vi "Convert LIN frames to Trace log.vi"(11 "lin frames in":T1[](array[typedef]) {"event ID" format="%x"; "payload" format="%x"; "timestamp" format="%<%.7X\n%x>T"; "type" items=["LIN Data"=64, "LIN Bus Error"=65, "LIN No Response"=66, "Delay"=224, "Log Trigger"=225, "Start Trigger"=226]; "identifier" format="%x"}) -> (3 "trace out":string[][](array[string]))   [LabVIEW 2025, in "CAN-LIN Raw Bus Capture.lvclass"]
uses:
  CAN-LIN Raw Bus Capture.lvclass
  <vilib>/xnet/xnet.llb/XNET Frame LIN.ctl
  <vilib>/xnet/xnet.llb/XNET Frame Type LIN.ctl
  CAN-LIN Raw Bus Capture.lvclass/CAN-LIN Raw Bus Capture.ctl
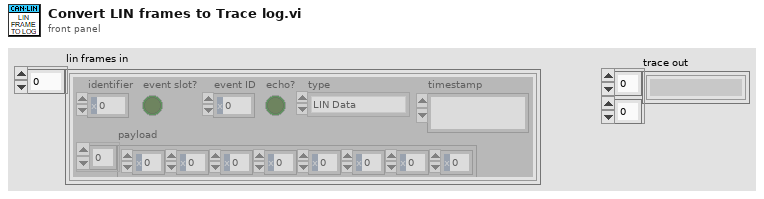
[diagram p1: front panel]
types:
  T1 = typedef "XNET Frame LIN.ctl" = cluster{"timestamp":timestamp, "payload":u8[], "identifier":u32, "type":T2, "event ID":u8, "event slot?":bool, "echo?":bool}
  T2 = typedef "XNET Frame Type LIN.ctl" = u8
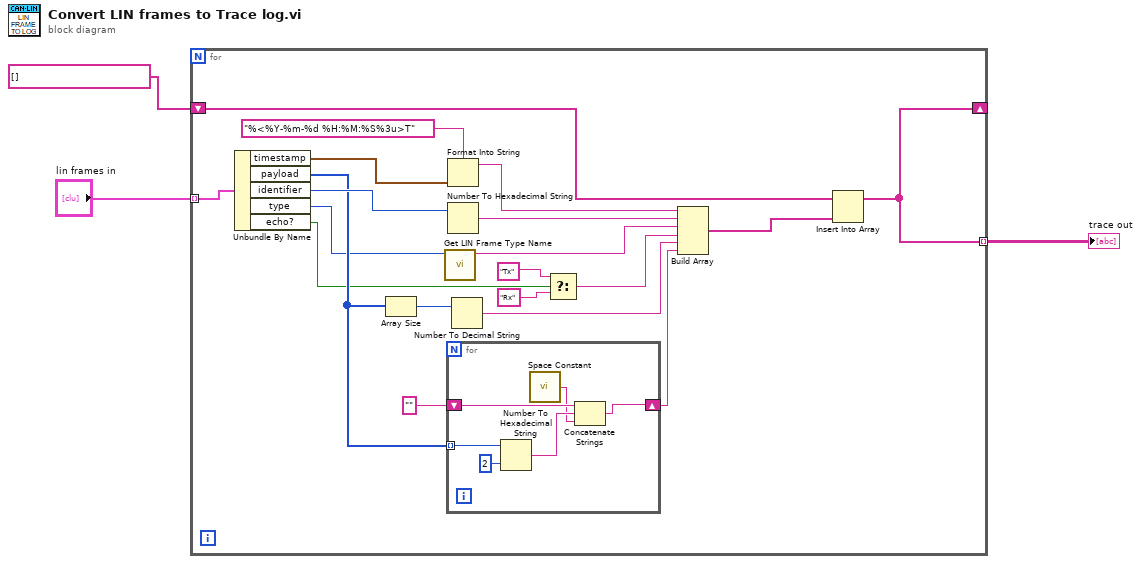
[diagram p0: block diagram]
diagram:
  n1 = for {
    tunnel: "lin frames in" -> [w23] mode=indexing
    tunnel: [w15] -> w3 mode=indexing
    shift-right: [w15] -> _
    shift-left: string[] [] ("Display") -> [w16]
    n2 = Unbundle By Name(w23) -> ("timestamp"=w19:timestamp, "payload"=w13:u8[], "identifier"=w22:u32, "type"=w11:T2, "echo?"=w5:bool)
    n3 = Array Size(array=w13) -> (size(s)=w14:i32)
    n4 = call "Get LIN Frame Type Name.vi"("lin frame type id"=w11) -> ("lin frame type name"=w10:string)  [unwired: 10 in]
    n5 = for {
      tunnel: w13 -> [w29] mode=indexing
      shift-right: [w26] -> w9
      shift-left: "" ("format string") -> [w28]
      n6 = Number To Hexadecimal String(1:i16 2 ("width (-)"), 2:w29) -> (0:w27:string)
      n7 = call <vilib>:"Space Constant.vi"() -> ("String"=w24:string)
      n8 = Concatenate Strings(w28, w27, w24) -> (w26:string)
    }
    n9 = Format Into String(format string="%<%Y-%m-%d %H:%M:%S%3u>T", w19) -> (resulting string=w18:string)  [unwired: 2 in, 1 out]
    n10 = Number To Hexadecimal String(2:w22) -> (0:w21:string)  [unwired: 1 in]
    n11 = Number To Decimal String(number=w14) -> (decimal integer string=w8:string)  [unwired: 1 in]
    n12 = Select(t="Tx" ("format string"), s=w5, f="Rx" ("format string")) -> (s? t:f=w4:string)
    n13 = Build Array(w18, w21, w10, w4, w8, w9) -> (w20:string[])
    n14 = Insert Into Array(array=w16, new element=w20) -> (w15:string[])  [unwired: 1 in]
  }
  "trace out" <- w3
